vi "DrawToolGradient.vi"(9 "Width":i32) -> (3 "Background":picture)   [LabVIEW 2020, in "Gviewer.lvclass"]
doc: "Plot Gradient backgrount on toolbar"
uses:
  Gviewer.lvclass
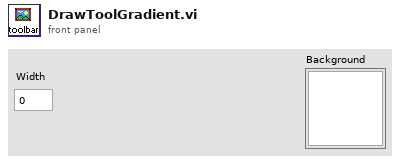
[diagram p1: front panel]
types:
  T1 = typedef "imagedata.ctl" = cluster{"image type":i32, "image depth":i32, "image":u8[], "mask":u8[], "colors":u32[], "Rectangle":cluster{"left":i16, "top":i16, "right":i16, "bottom":i16}}
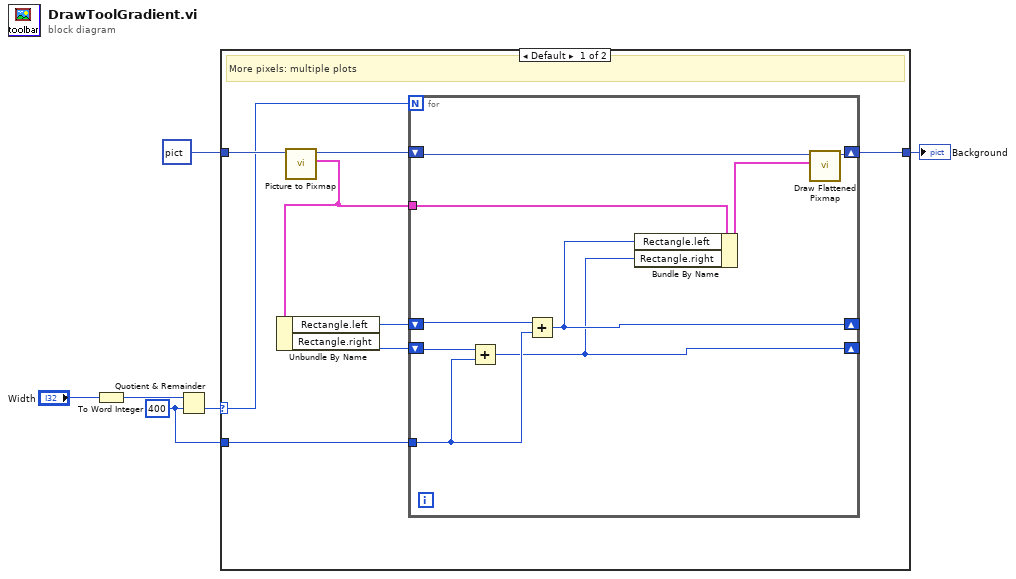
[diagram p0: block diagram]
diagram:
  w2 = i16 400 ("y")
  n1 = To Word Integer(number="Width") -> (16bit integer=w1:i16)
  n2 = Quotient & Remainder(x=w1, y=w2) -> (floor(x/y)=w5:i16)  [unwired: 1 out]
  n3 = case shown="Default" w5 {
    selector: w5 -> [w7 _]
    tunnel: picture bytes[42270] ("2D Picture") -> [w14 w24]
    tunnel: [w8 w24] -> w3
    tunnel: w2 -> [w9 _]
    frame Default {
      # "More pixels: multiple plots"
      n4 = call <vilib>:"Picture to Pixmap.vi"("picture"=w14) -> ("image data"=w12:T1, "new picture"=w13:picture)  [unwired: 9 in]
      n5 = Unbundle By Name(w12) -> ("Rectangle.left"=w11:i16, "Rectangle.right"=w10:i16)
      n6 = for {
        N: w7 -> [_]
        shift-right: [w19] -> w8
        shift-left: w13 -> [w20]
        tunnel: w12 -> [w18]
        shift-right: [w16] -> _
        shift-left: w11 -> [w23]
        shift-right: [w15] -> _
        shift-left: w10 -> [w22]
        tunnel: w9 -> [w21]
        n7 = Add(x=w22, y=w21) -> (x+y=w15:i16)
        n8 = Add(x=w23, y=w21) -> (x+y=w16:i16)
        n9 = Bundle By Name(cluster=w18, "Rectangle.left"=w16, "Rectangle.right"=w15) -> (w17:T1)
        n10 = call <vilib>:"Draw Flattened Pixmap.vi"("image data"=w17, "picture"=w20) -> ("new picture"=w19:picture)  [unwired: 7 in]
      }
    }
    frame 0 {
      # "0 - 400 pixels"
    }
  }
  "Background" <- w3
